vi "Flatten2DArray.vi"(8 "error in (no error)":errorcluster, 11 "2D Array In":i8[][](array[numeric])) -> (0 "error out":errorcluster, 3 "1D Array Out":i8[](array[numeric]))   [LabVIEW 2020]
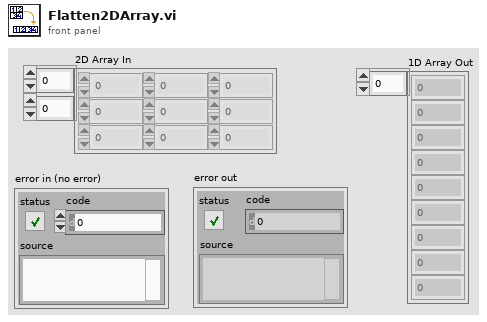
[diagram p1: front panel]
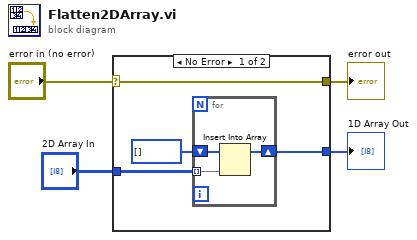
[diagram p0: block diagram]
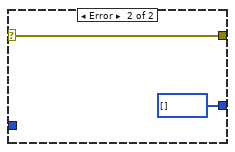
[diagram p2: hidden frame]
diagram:
  n1 = case shown="No Error" "error in (no error)" {
    selector: "error in (no error)" -> [w5 w13]
    tunnel: [w5 w13] -> w3
    tunnel: "2D Array In" -> [w8 _]
    tunnel: [w6 i8[] [] ("1D Array Out")] -> w1
    frame No Error {
      n2 = for {
        tunnel: w8 -> [w9] mode=indexing
        shift-right: [w10] -> w6
        shift-left: i8[] [] ("1D Array Out") -> [w11]
        n3 = Insert Into Array(array=w11, new element=w9) -> (w10:i8[])  [unwired: 1 in]
      }
    }
    frame Error {
    }
  }
  "error out" <- w3
  "1D Array Out" <- w1
